vi "read user data.vi"(8 "error in (no error)":errorcluster, 11 "file name":string) -> (0 "error out":errorcluster, 1 "values":string[][](array[string]), 2 "key names":string[][](array[string]), 3 "LABEL":string[][](array[string]))   [LabVIEW 2024]
uses:
  <vilib>/Utility/config.llb/Read Key (String).vi
  <vilib>/Utility/config.llb/NI_LVConfig.lvlib
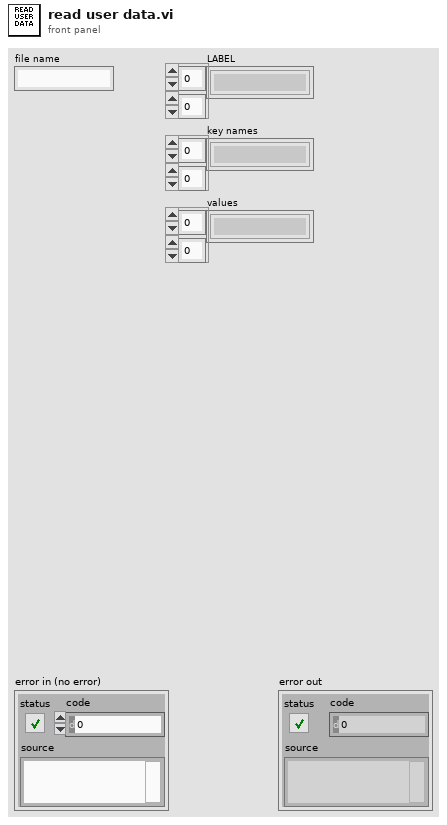
[diagram p1: front panel]
types:
  T1 = typedef "NI_LVConfig.lvlib/Config Data RefNum.ctl" = refnum<k1>
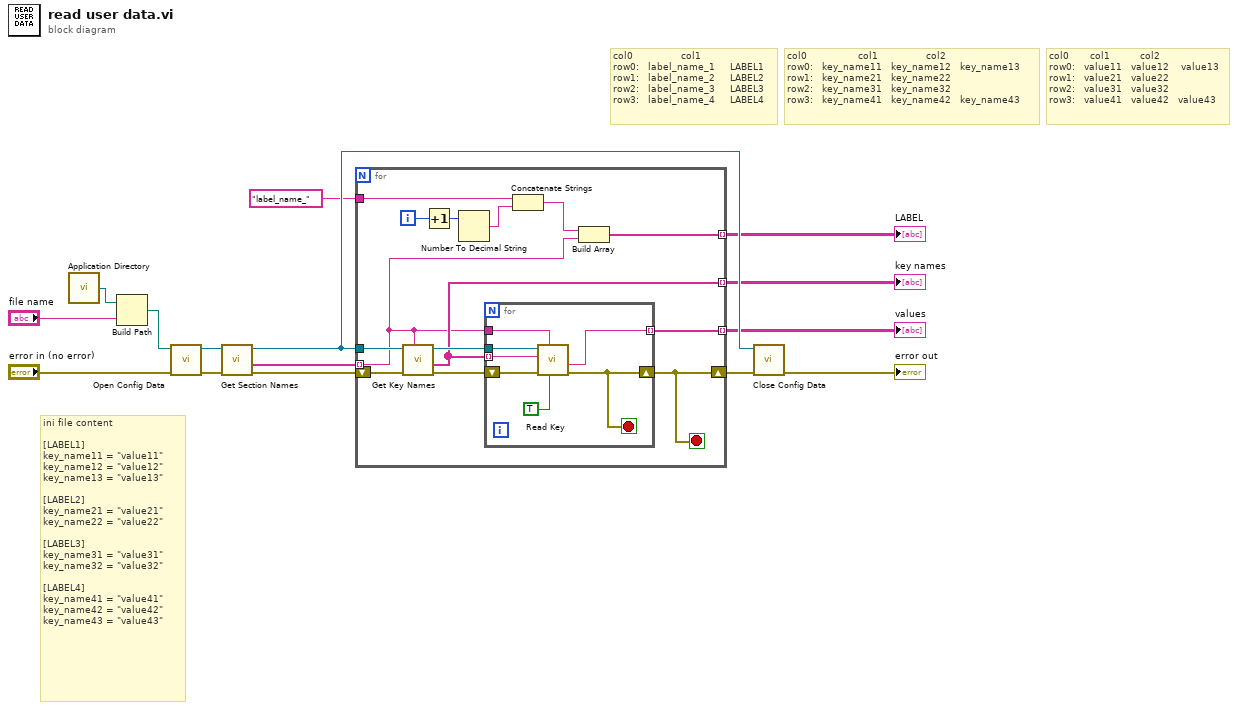
[diagram p0: block diagram]
diagram:
  # "col0       col1          col2\nrow0:   value11   value12    value13\nrow1:   value21   value22\nrow2:   value31   value32\nrow3:   value41   value42   value43"
  # "col0                 col1                col2\nrow0:   key_name11   key_name12   key_name13\nrow1:   key_name21   key_name22 \nrow2:   key_name31   key_name32  \nrow3:   key_name41   key_name42   key_name43"
  # "col0                col1\nrow0:   label_name_1     LABEL1\nrow1:   label_name_2     LABEL2\nrow2:   label_name_3     LABEL3\nrow3:   label_name_4     LABEL4"
  # "ini file content\n\n[LABEL1]\nkey_name11 = \"value11\"\nkey_name12 = \"value12\" \nkey_name13 = \"value13\"\n\n[LABEL2]\nkey_name21 = \"value21\"\nkey_name22 = \"value22\"  \n\n[LABEL3]\nkey_name31 = \"value31\"\nkey_name32 = \"value32\"    \n\n[LABEL4]\nkey_name41 = \"value41\"\nkey_name42 = \"value42\"    \nkey_name43 = \"value43\""
  n1 = call <vilib>:"Application Directory.vi"() -> ("Application Directory"=w8:path)
  n2 = Build Path(base path=w8, name or relative path="file name") -> (appended path=w10:path)
  n3 = call <vilib>:"Open Config Data.vi"("error in (no error)"="error in (no error)", "configuration file path"=w10) -> ("error out"=w13:errorcluster, "refnum"=w12:T1)  [unwired: 7 in, 1 out]
  n4 = call <vilib>:"Get Section Names.vi"("error in (no error)"=w13, "refnum"=w12) -> ("error out"=w14:errorcluster, "section names"=w6:string[], "refnum out"=w15:T1)  [unwired: 7 in]
  n5 = for {
    tunnel: w15 -> [w29]
    tunnel: w6 -> [w17] mode=indexing
    shift-right: [w25] -> w2
    shift-left: w14 -> [w28]
    tunnel: "label_name_" -> [w22]
    tunnel: [w20] -> w5 mode=indexing
    tunnel: [w19] -> w4 mode=indexing
    tunnel: [w16] -> w3 mode=indexing
    i -> [w23]
    stop <- w25 stop-if-true
    n6 = call <vilib>:"Get Key Names.vi"("section"=w17, "error in (no error)"=w28, "refnum"=w29) -> ("error out"=w27:errorcluster, "key names"=w20:string[], "refnum out"=w26:T1)  [unwired: 5 in, 1 out]
    n7 = Increment(x=w23) -> (x+1=w24:i32)
    n8 = Number To Decimal String(number=w24) -> (decimal integer string=w21:string)  [unwired: 1 in]
    n9 = for {
      shift-right: [w31] -> w25
      shift-left: w27 -> [w36]
      tunnel: w20 -> [w32] mode=indexing
      tunnel: w26 -> [w35]
      tunnel: w17 -> [w34]
      tunnel: [w33] -> w19 mode=indexing
      stop <- w31 stop-if-true
      n10 = call-poly <vilib>:"Read Key.vi"("read raw string? (F)"=TRUE, "section"=w34, "error in (no error)"=w36, "key"=w32, "refnum"=w35) -> ("error out"=w31:errorcluster, "value"=w33:string)  [unwired: 3 in, 2 out]
    }
    n11 = Concatenate Strings(w22, w21) -> (w18:string)
    n12 = Build Array(w18, w17) -> (w16:string[])
  }
  "LABEL" <- w3
  "key names" <- w5
  "values" <- w4
  n13 = call <vilib>:"Close Config Data.vi"("error in (no error)"=w2, "refnum"=w15) -> ("error out"=→"error out":errorcluster)  [unwired: 8 in, 1 out]
